vi "MHL Queue Ref Holder.vi"(8 "error in":errorcluster, 11 "Message Queue In":refnum<queue>) -> (0 "error out":errorcluster, 3 "Input Message Queue":refnum<queue>)   [LabVIEW 2015]
doc: "Holds UI queue reference to enqueue messages without wiring"
uses:
  Message Queue/Message Cluster.ctl
  Message Queue/Message Queue.lvlib
panel:
  in  "Action":enum16{"GET", "SET"}(ring)
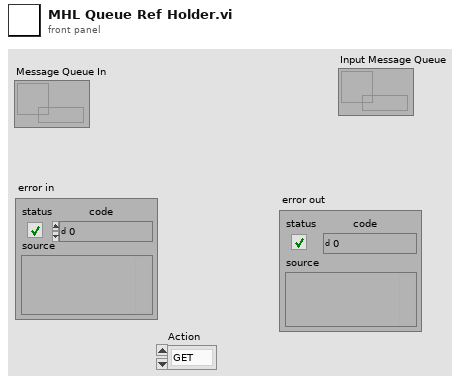
[diagram p1: front panel]
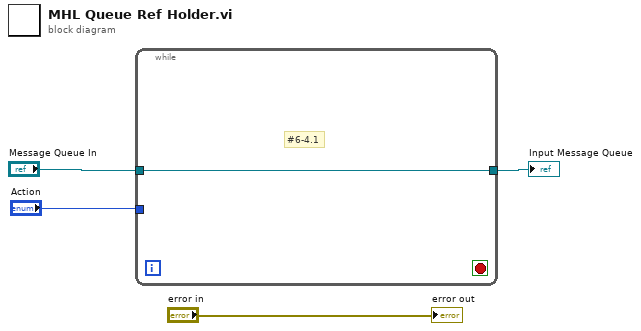
[diagram p0: block diagram]
diagram:
  n1 = while {
    tunnel: "Message Queue In" -> [w5]
    tunnel: [w5] -> w3
    tunnel: "Action" -> [_]
    stop <- _ stop-if-true
    # "#6-4.1"
  }
  "Input Message Queue" <- w3
  "error out" <- "error in"
